vi "Handle Actor Core Events.vi"(8 "error in (no error)":errorcluster, 11 "ActorAutoRegistration in":refnum<class "ActorAutoRegistration.lvclass">) -> (0 "error out":errorcluster)   [LabVIEW 2015, in "ActorAutoRegistration.lvlib" / "ActorAutoRegistration.lvclass"]
uses:
  ActorAutoRegistration.lvclass
  ActorAutoRegistration.lvclass/ActorAutoRegistration.ctl
  ActorAutoRegistration Messages/PanelCloseMsg/PanelCloseMsg.lvclass
  ActorAutoRegistration Messages/ValueChangeMsg/ValueChangeMsg.lvclass
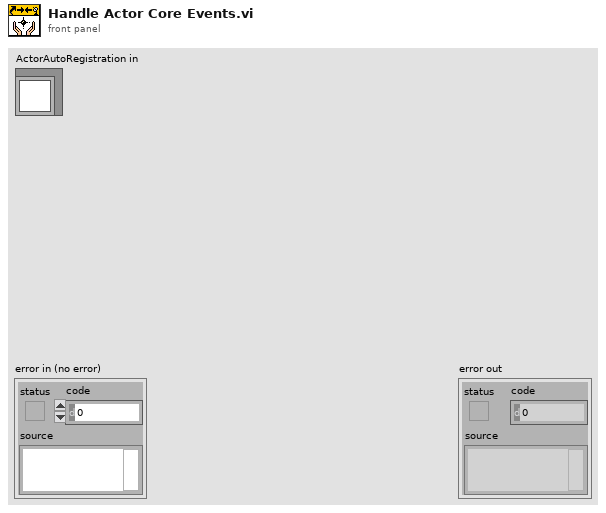
[diagram p1: front panel]
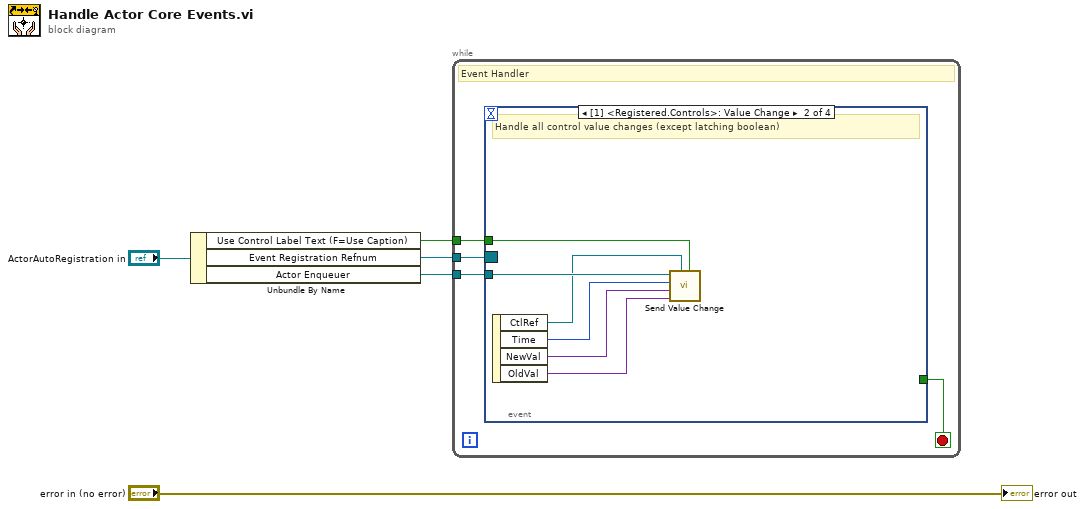
[diagram p0: block diagram]
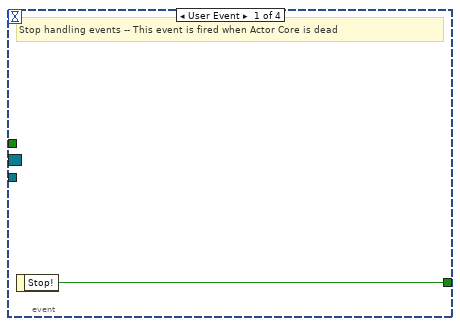
[diagram p2: hidden frame]
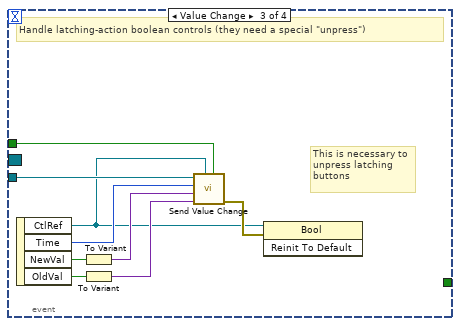
[diagram p3: hidden frame]
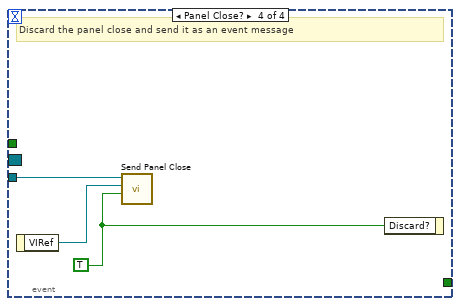
[diagram p4: hidden frame]
diagram:
  n1 = Unbundle By Name("ActorAutoRegistration in") -> ("Use Control Label Text (F=Use Caption)"=w1:bool, "Event Registration Refnum"=w3:refnum<event-registration>, "Actor Enqueuer"=w2:refnum<class "Message Enqueuer.lvclass">)
  n2 = while {
    tunnel: w3 -> [w9]
    tunnel: w2 -> [w7]
    tunnel: w1 -> [w6]
    stop <- w8 stop-if-true
    # "Event Handler"
    n3 = event shown="[1] <Registered.Controls>: Value Change" {
      selector: w9 -> [_ _ _ _]
      dyn-events: _ -> [_ _ _ _]
      timeout: _ -> [_ _ _ _]
      tunnel: [w10 _ _ _] -> w8
      tunnel: w7 -> [_ w16 w25 w28]
      tunnel: w6 -> [_ w11 w17 _]
      event User Event {
        # "Stop handling events -- This event is fired when Actor Core is dead"
        n4 = event-data() -> ("Stop!"=w10:bool)  [unwired: 1 in]
      }
      event Value Change {
        # "Handle all control value changes (except latching boolean)"
        n5 = event-data() -> ("CtlRef"=w12:refnum<vi>, "Time"=w15:u32, "NewVal"=w14:variant, "OldVal"=w13:variant)  [unwired: 1 in]
        n6 = call "Send Value Change.vi"("Use Label Text (F=Use Caption)"=w11, "Ctl Refnum"=w12, "New Value"=w13, "Old Value"=w14, "Time"=w15, "Message Enqueuer in"=w16) -> ()  [unwired: 5 in, 1 out]
      }
      event Value Change {
        # "This is necessary to\nunpress latching\nbuttons"
        # "Handle latching-action boolean controls (they need a special \"unpress\")"
        n7 = event-data() -> ("CtlRef"=w18:refnum<vi>, "Time"=w24:u32, "NewVal"=w23:bool, "OldVal"=w22:bool)  [unwired: 1 in]
        n8 = To Variant(anything=w23) -> (Variant=w20:variant)
        n9 = To Variant(anything=w22) -> (Variant=w21:variant)
        n10 = call "Send Value Change.vi"("Use Label Text (F=Use Caption)"=w17, "Ctl Refnum"=w18, "New Value"=w21, "Old Value"=w20, "Time"=w24, "Message Enqueuer in"=w25) -> ("error out"=w19:errorcluster)  [unwired: 5 in]
        n11 = invoke class="Bool" method="Reinit To Default"(reference=w18, error in=w19) -> ()  [unwired: 1 in, 3 out]
      }
      event Panel Close? {
        w26 = TRUE ("Discarded?")
        # "Discard the panel close and send it as an event message"
        n12 = event-data() -> ("VIRef"=w27:refnum<vi>)  [unwired: 1 in]
        n13 = call "Send Panel Close.vi"("Discarded?"=w26, "VI Refnum"=w27, "Message Enqueuer in"=w28) -> ()  [unwired: 8 in, 1 out]
        n14 = event-data("Discard?"=w26) -> ()  [unwired: 1 in, 1 out]
      }
    }
  }
  "error out" <- "error in (no error)"
